vi "求阶乘（U64).vi"(1 "Num":i32=100) -> (0 "Fract":u64)   [LabVIEW 2012]
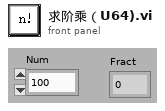
[diagram p1: front panel]
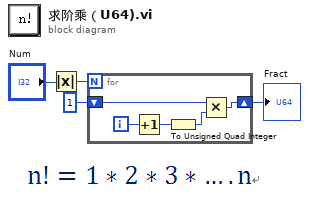
[diagram p0: block diagram]
diagram:
  n1 = Absolute Value(x="Num") -> (abs(x)=w3:i32)
  n2 = for {
    N: w3 -> [_]
    shift-right: [w6] -> w1
    shift-left: u64 1 -> [w7]
    i -> [w9]
    n3 = Increment(x=w9) -> (x+1=w8:i32)
    n4 = To Unsigned Quad Integer(1:w8) -> (0:w5:u64)
    n5 = Multiply(x=w7, y=w5) -> (x*y=w6:u64)
  }
  "Fract" <- w1
